vi "Change_Coordinates.vi"(10 "Ball Coordinates":cluster{"x":sgl, "y":sgl}, 11 "Plate coordinates":sgl[](array[numeric])) -> (3 "Array":sgl[](array[numeric]))   [LabVIEW 2021]
doc: "Takes absolute ball and plate xy coordinates and computes new ball coordinates. The origin is at the center of the plate, x and y direction are taken parallel to x and y direction of the servo base units (see VI icon). Returns 0 if ball is not found"
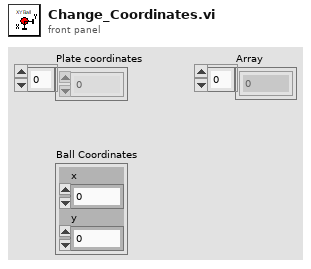
[diagram p1: front panel]
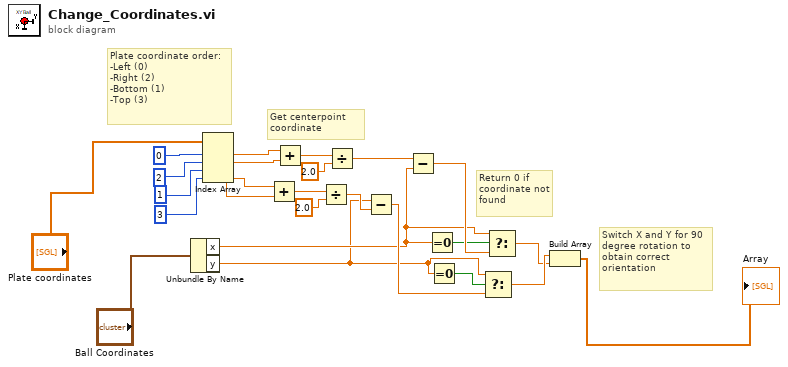
[diagram p0: block diagram]
diagram:
  # "Switch X and Y for 90 degree rotation to obtain correct orientation"
  # "Return 0 if coordinate not found"
  # "Get centerpoint \ncoordinate"
  # "Plate coordinate order:\n-Left (0)\n-Right (2)\n-Bottom (1)\n-Top (3)"
  n1 = Unbundle By Name("Ball Coordinates") -> ("x"=w20:sgl, "y"=w2:sgl)
  n2 = Index Array(array="Plate coordinates", index #1=0 ("index"), index #2=2 ("index"), index #3=1 ("index"), index #4=3 ("index")) -> (element #1=w10:sgl, element #2=w11:sgl, element #3=w16:sgl, element #4=w17:sgl)
  n3 = Add(x=w16, y=w17) -> (x+y=w14:sgl)
  n4 = Add(x=w10, y=w11) -> (x+y=w12:sgl)
  n5 = Divide(x=w14, y=sgl 2.0) -> (x/y=w3:sgl)
  n6 = Divide(x=w12, y=sgl 2.0) -> (x/y=w18:sgl)
  n7 = Subtract(x=w2, y=w3) -> (x-y=w23:sgl)
  n8 = Subtract(x=w18, y=w20) -> (x-y=w21:sgl)
  n9 = Equal To 0?(x=w20) -> (x = 0?=w19:bool)
  n10 = Equal To 0?(x=w2) -> (x = 0?=w22:bool)
  n11 = Select(t=w2, s=w22, f=w23) -> (s? t:f=w5:sgl)
  n12 = Select(t=w20, s=w19, f=w21) -> (s? t:f=w4:sgl)
  n13 = Build Array(w5, w4) -> (→"Array":sgl[])
